vi "Configure Channel Display IO.vi"(0 "VISA resource name":refnum<visa-resource-name>, 1 "Lower Zone (0)":i32 min=0 max=95 step=1, 2 "Upper Zone (100)":i32=100 min=5 max=100 step=1, 5 "IO Channel (0001)":string="0001", 7 "Color":cluster{"R":i32, "G":i32, "B":i32} {"B" min=0 max=255 step=1; "G" min=0 max=255 step=1; "R" min=0 max=255 step=1}, 11 "error in (no error)":errorcluster, 12 "Scale Position (1: 1)":i32(ring)=1 items=["Off", "1", "2", "3", "4", "5", "6", "7", "8", "9", "10"], 13 "Scale Division (10: 10)":i32(ring)=10 items=["4"=4, "5"=5, "6"=6, "7"=7, "8"=8, "9"=9, "10"=10, "11"=11, "12"=12, "C10"=13]) -> (4 "VISA resource name out":refnum<visa-resource-name>, 6 "IO Channel":string, 15 "error out":errorcluster)   [LabVIEW 2020, in "Yokogawa GX Series.lvlib"]
doc: "Sets the zone, channel display color and the scale.\n\nCommands: SColorIO, SZoneIO, SScaleIO\n\nNote: This VI doesn't send SScaleIO command when the instrument is GM10."
uses:
  <instrlib>/Yokogawa GX Series/Yokogawa GX Series.lvlib
panel:
  # "%"
  # "%"
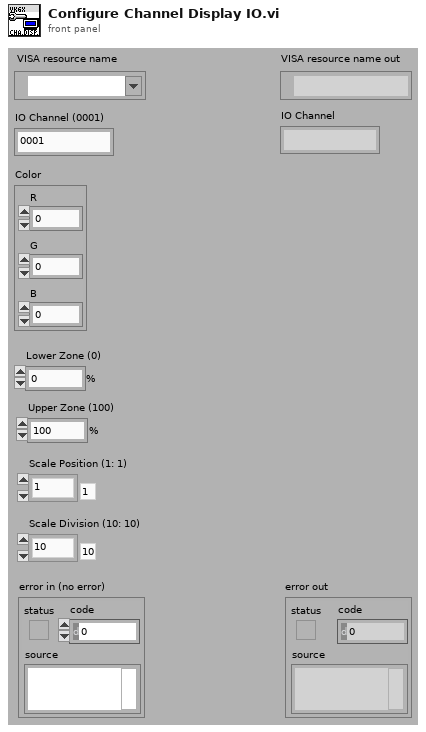
[diagram p1: front panel]
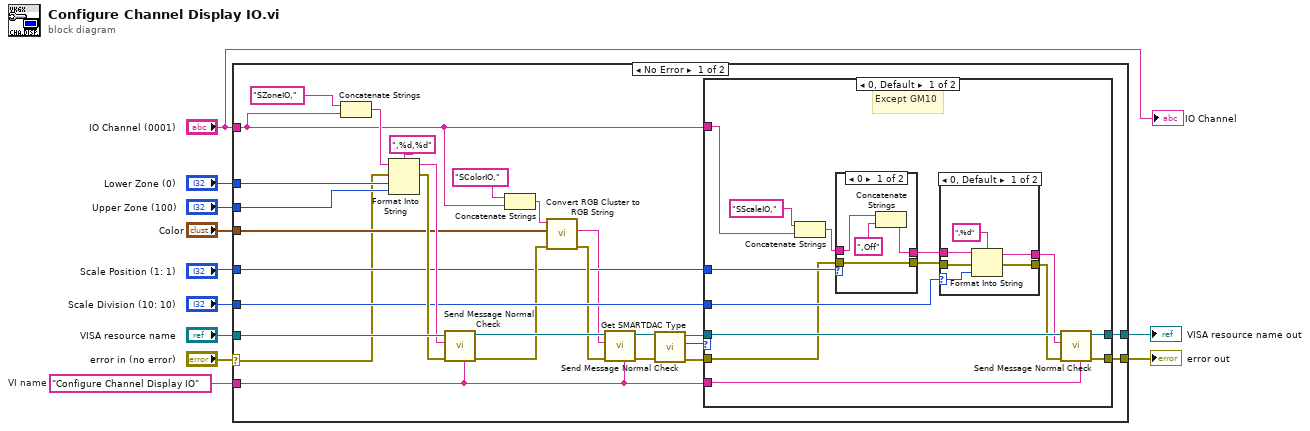
[diagram p0: block diagram]
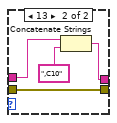
[diagram p2: hidden frame]
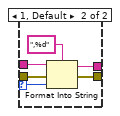
[diagram p3: hidden frame]
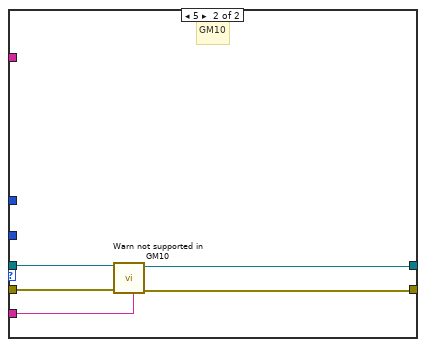
[diagram p4: hidden frame]
diagram:
  w10 = "Configure Channel Display IO"  # VI name
  n1 = case shown="No Error" "error in (no error)" {
    selector: "error in (no error)" -> [w18 w78]
    tunnel: "VISA resource name" -> [w34 w79]
    tunnel: w10 -> [w31 _]
    tunnel: "Lower Zone (0)" -> [w30 _]
    tunnel: "Upper Zone (100)" -> [w29 _]
    tunnel: "Scale Division (10: 10)" -> [w27 _]
    tunnel: [w26 w79] -> w6
    tunnel: [w25 w78] -> w5
    tunnel: "Color" -> [w24 _]
    tunnel: "Scale Position (1: 1)" -> [w20 _]
    tunnel: "IO Channel (0001)" -> [w19 _]
    frame No Error {
      n2 = Concatenate Strings("SZoneIO,", w19) -> (w36:string)
      n3 = Format Into String(format string=",%d,%d", initial string=w36, error in=w18, w30, w29) -> (resulting string=w33:string, error out=w32:errorcluster)
      n4 = call <instrlib>:"Send Message Normal Check.vi"("Source (\"\")"=w31, "error in (no error)"=w32, "Send Message (\"\")"=w33, "VISA resource name"=w34) -> ("error out"=w23:errorcluster, "VISA resource name out"=w28:refnum<visa-resource-name>)  [unwired: 2 in, 4 out]
      n5 = Concatenate Strings("SColorIO,", w19) -> (w21:string)
      n6 = call <instrlib>:"Convert RGB Cluster to RGB String.vi"("error in (no error)"=w23, "RGB"=w24, "Initial String"=w21) -> ("error out"=w22:errorcluster, "RGB String"=w17:string)  [unwired: 7 in]
      n7 = call <instrlib>:"Send Message Normal Check.vi"("Source (\"\")"=w31, "error in (no error)"=w22, "Send Message (\"\")"=w17, "VISA resource name"=w28) -> ("error out"=w15:errorcluster, "VISA resource name out"=w16:refnum<visa-resource-name>)  [unwired: 2 in, 4 out]
      n8 = call <instrlib>:"Get SMARTDAC Type.vi"("error in (no error)"=w15, "VISA resource name"=w16) -> ("error out"=w13:errorcluster, "SMARTDAC+ Type"=w12:u16, "VISA resource name out"=w14:refnum<visa-resource-name>)  [unwired: 7 in]
      n9 = case shown="0, Default" w12 {
        tunnel: w31 -> [w52 w73]
        tunnel: w27 -> [w44 _]
        tunnel: [w51 w75] -> w26
        tunnel: [w50 w74] -> w25
        tunnel: w14 -> [w47 w77]
        tunnel: w13 -> [w39 w76]
        tunnel: w20 -> [w45 _]
        tunnel: w19 -> [w46 _]
        frame 0, Default {
          # "Except GM10"
          n10 = Concatenate Strings("SScaleIO,", w46) -> (w43:string)
          n11 = case shown="0" w45 {
            selector: w45 -> [_ w69]
            tunnel: w39 -> [w63 w67]
            tunnel: [w63 w71] -> w48
            tunnel: [w64 w70] -> w42
            tunnel: w43 -> [w65 w68]
            frame 0 {
              n12 = Concatenate Strings(w65, ",Off") -> (w64:string)
            }
            frame 1, Default {
              n13 = Format Into String(format string=",%d" ("形式文字列"), initial string=w68, error in=w67, w69) -> (resulting string=w70:string, error out=w71:errorcluster)
            }
          }
          n14 = case shown="0, Default" w44 {
            selector: w44 -> [w54 _]
            tunnel: w48 -> [w57 w62]
            tunnel: [w56 w62] -> w41
            tunnel: [w55 w59] -> w40
            tunnel: w42 -> [w53 w61]
            frame 0, Default {
              n15 = Format Into String(format string=",%d" ("形式文字列"), initial string=w53, error in=w57, w54) -> (resulting string=w55:string, error out=w56:errorcluster)
            }
            frame 13 {
              n16 = Concatenate Strings(w61, ",C10") -> (w59:string)
            }
          }
          n17 = call <instrlib>:"Send Message Normal Check.vi"("Source (\"\")"=w52, "error in (no error)"=w41, "Send Message (\"\")"=w40, "VISA resource name"=w47) -> ("error out"=w50:errorcluster, "VISA resource name out"=w51:refnum<visa-resource-name>)  [unwired: 2 in, 4 out]
        }
        frame 5 {
          # "GM10"
          n18 = call <instrlib>:"Warn not supported in GM10.vi"("Source (\"\")"=w73, "error in (no error)"=w76, "VISA resource name"=w77) -> ("error out"=w74:errorcluster, "VISA resource name out"=w75:refnum<visa-resource-name>)  [unwired: 7 in]
        }
      }
    }
    frame Error {
    }
  }
  "error out" <- w5
  "VISA resource name out" <- w6
  "IO Channel" <- "IO Channel (0001)"
